vi "tearDown.vi"(8 "error in (no error)":errorcluster, 11 "reference in":refnum<class "List_Delegations.lvclass">) -> (0 "error out":errorcluster, 3 "reference out":refnum<class "List_Delegations.lvclass">)   [LabVIEW 2009, in "List_Delegations.lvclass"]
doc: "tearDown runs after the test method has completed. Use this method to clean up any operations or references that were opened by setUp or the test method. Unit tests should be independent of other unit tests so this VI should ensure that the next test can run in a 'clean' test environment."
uses:
  List_Delegations.lvclass
  List_Delegations.lvclass/List_Delegations.ctl
  source/Lists/List/List.lvclass
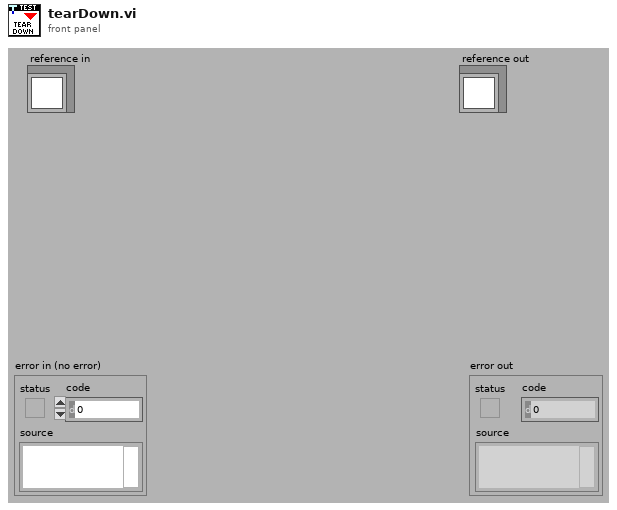
[diagram p1: front panel]
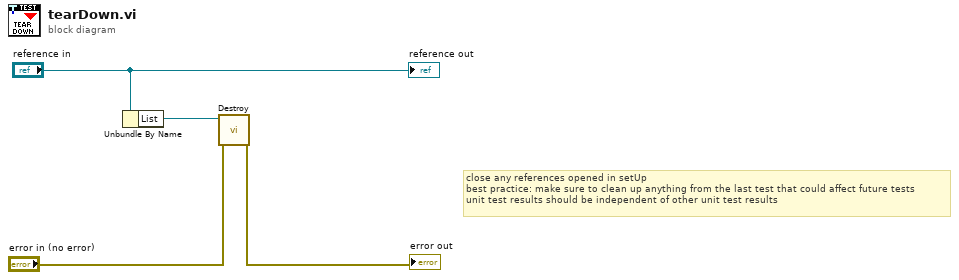
[diagram p0: block diagram]
diagram:
  # "close any references opened in setUp\nbest practice: make sure to clean up anything from the last test that could affect future tests\nunit test results should be independent of other unit test results"
  n1 = Unbundle By Name("reference in") -> ("List"=w3:refnum<class "List.lvclass">)
  n2 = call-dynamic "Destroy.vi"("error in (no error)"="error in (no error)", "List in"=w3) -> ("error out"=→"error out":errorcluster)  [unwired: 9 in]
  "reference out" <- "reference in"
